vi "RT Main IMAQdx.vi"() -> ()   [LabVIEW 2017]
doc: "The myRIO Custom FPGA Project template acquires button data from the onboard button and displays the button value on a Boolean indicator. The SYS.RDY indicator shows the FPGA status."
uses:
  Controls/Image Size.ctl
  <vilib>/userdefined/High Color/IMAQdx.ctl
  <vilib>/FPGAPlugInAG/Dynamic/niLvFpga_Close_Dynamic.vi
  <vilib>/rvi/errors/niLvFpgaAdjustHostInterfaceError.vi
  <vilib>/Utility/error.llb/Error Cluster From Error Code.vi
  <vilib>/FPGAPlugInAG/Dynamic/niLvFpga_Run_Dynamic.vi
  <vilib>/myRIO/Common/Instrument Driver Framework/Utilities/vis/FPGA Ref Manager.vi
  <vilib>/myRIO/Common/Instrument Driver Framework/Utilities/vis/Ref Counter.vi
  <vilib>/rvi/interface/common/niFpgaCacheSessionInfoDynamic.vi
  <vilib>/rvi/interface/RandomDataEmulation/nirviRandomDataOpen.vi
  <vilib>/rvi/interface/nirviCloseFPGA/nirviCloseFPGA.xnode
  <vilib>/rvi/interface/nirviMethod/nirviMethod.xnode
  <vilib>/rvi/interface/nirviOpenFPGA/nirviOpenFPGA.xnode
  FPGA Main Image Processing.vi
  <vilib>/myRIO/Instrument Drivers/Utilities/Utilities.lvlib
  <vilib>/rvi/errors/niLvFpgaMergeErrorWithErrorCode.vi
  <vilib>/vision/NI_Vision_Development_Module.lvlib
  <vilib>/vision/driver/NI_Vision_Acquisition_Software.lvlib
  <vilib>/FPGAPlugInAG/Dynamic/niLvFpga_ReadFifo_Dynamic.vi
  <vilib>/FPGAPlugInAG/Dynamic/niLvFpga_WriteFifo_Dynamic.vi
  <vilib>/FPGAPlugInAG/Dynamic/niLvFpga_Reset_Dynamic.vi
  FPGA Bitfiles/SoCImageProcessi_FPGATarget_FPGAMainImagePro_62bwVpL48zU.lvbitx
  <vilib>/FPGAPlugInAG/myRIO-1900/niLvFpga_Open_myRIO-1900.vi
  <vilib>/rvi/interface/common/dynamic/niFpgaDynamicAddResources.vi
panel:
  out "Image Out":T1(plugin-control)
  out "Image In":T1(plugin-control)
  in  "Live":bool
  in  "Timeout":i32=2000
  out "FPS":dbl format="%#_3f"
  out "error out":errorcluster
  in  "Stop":bool
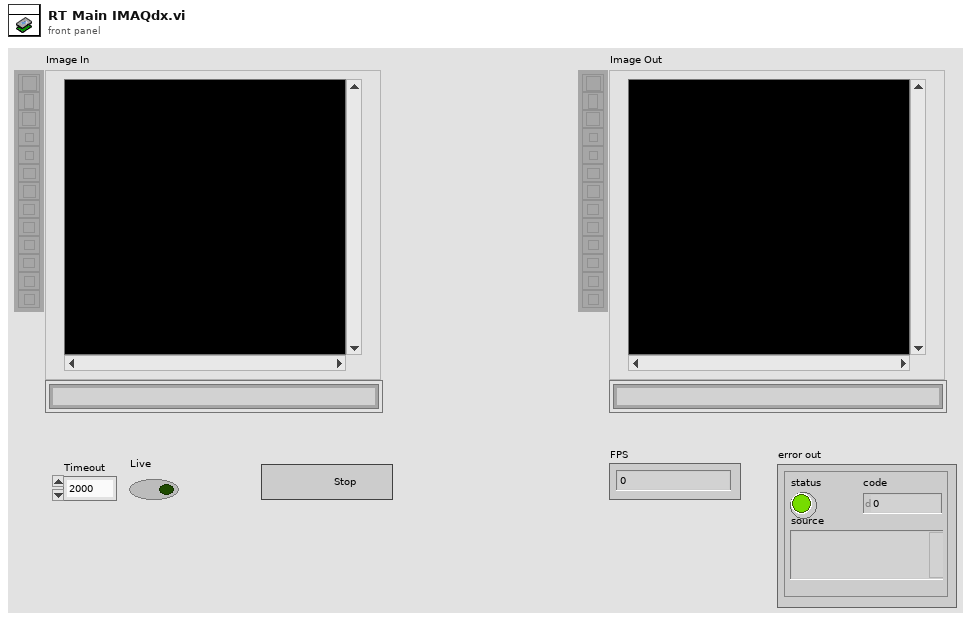
[diagram p1: front panel]
types:
  T1 = typedef "IMAQ Image.ctl" = refnum<image>
  T2 = typedef "Image Size.ctl" = cluster{"Rows (X)":u16, "Colums (Y)":u16}
  T3 = typedef "IMAQdx.ctl" = refnum<k21>
  T4 = typedef "Image Type" = u32
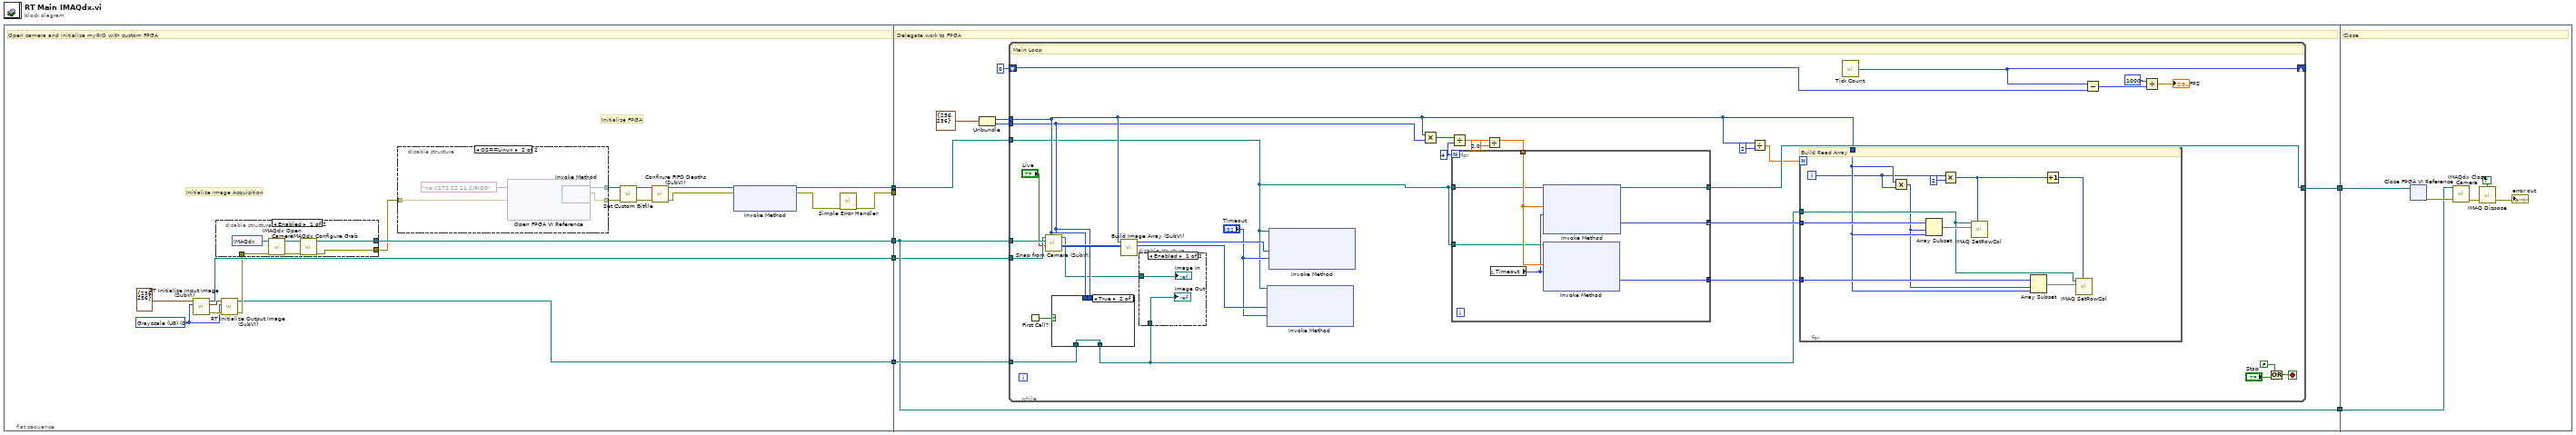
[diagram p0: block diagram]
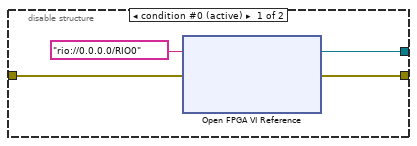
[diagram p3: hidden frame]
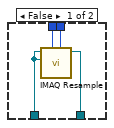
[diagram p5: hidden frame]
diagram:
  n1 = flat-sequence {
    tunnel: [w19] -> w7
    tunnel: [w24] -> w5
    tunnel: [w23] -> w4
    tunnel: [w9] -> w3
    tunnel: [w8] -> w1
    tunnel: w7 -> [w46]
    tunnel: [w50] -> w6
    tunnel: w5 -> [w44]
    tunnel: w4 -> [w43]
    tunnel: w3 -> [_]
    tunnel: [w44] -> w2
    tunnel: w1 -> [w45]
    tunnel: w6 -> [w114]
    tunnel: w2 -> [w109]
    frame #0 {
      w20 = T4 0 items=["Grayscale (U8)", "Grayscale (I16)", "Grayscale (SGL)", "Complex (CSG)", "RGB (U32)", "HSL (U32)", "RGB (U64)", "Grayscale (U16)"] ("Image Type")
      # "Initialize FPGA"
      # "Initialize Image Acquisition"
      # "Open camera and initialize myRIO with custom FPGA"
      n2 = call "RT Initialize Input Image (SubVI).vi"("Image Type"=w20, "Image Size In"=T2 {"Rows (X)"=256, "Colums (Y)"=256} ("Image Size")) -> ("error out"=w22:errorcluster, "Input Image Size Out"=w18:T2, "Input Image Out"=w23:T1)  [unwired: 7 in]
      n3 = call "RT Initialize Output Image (SubVI).vi"("error in (no error)"=w22, "Image Type"=w20, "Image Size In"=w18) -> ("error out"=w21:errorcluster, "Output Image Out"=w19:T1)  [unwired: 7 in]
      n4 = disable-structure shown="Enabled" {
        disable-tunnel: [w28 _] -> w24
        disable-tunnel: w21 -> [w27 w32]
        disable-tunnel: [w26 w32] -> w16
        frame Enabled {
          n5 = call <vilib>:"IMAQdx Open Camera.vi"("error in"=w27, "Session In"=T3 "cam0") -> ("error out"=w30:errorcluster, "Session Out"=w29:T3)  [unwired: 8 in]
          n6 = call <vilib>:"IMAQdx Configure Grab.vi"("error in"=w30, "Session In"=w29) -> ("error out"=w26:errorcluster, "Session Out"=w28:T3)  [unwired: 8 in]
        }
        frame Disabled {
        }
      }
      n7 = disable-structure shown="OS==Linux" {
        disable-tunnel: [w35 w39] -> w25
        disable-tunnel: [w34 w40] -> w17
        disable-tunnel: w16 -> [w33 w41]
        frame condition #0 (active) {
          n8 = xnode "Open FPGA VI Reference"("error in"=w33, "resource name"=tag "rio://0.0.0.0/RIO0") -> ("FPGA VI Reference Out"=w34:refnum<k20>, "error out"=w35:errorcluster)
        }
        frame condition #1 {
          n9 = xnode "Open FPGA VI Reference"("error in"=w41, "resource name"=tag "rio://172.22.11.2/RIO0") -> ("FPGA VI Reference Out"=w38:refnum<k20>, "error out"=w37:errorcluster)
          n10 = xnode "Invoke Method"("FPGA VI Reference In"=w38, "error in"=w37) -> ("FPGA VI Reference Out"=w40:refnum<k20>, "error out"=w39:errorcluster)
        }
      }
      n11 = call <vilib>:"Set Custom Bitfile.vi"("error in (no error)"=w25, "Custom FPGA Reference In"=w17) -> ("error out"=w13:errorcluster, "Custom FPGA Reference Out"=w10:refnum<k20>)  [unwired: 8 in]
      n12 = call "Confirure FIFO Depths (SubVI).vi"("error in (no error)"=w13, "Refnum in"=w10) -> ("error out"=w11:errorcluster, "Refnum out"=w12:refnum<k20>)  [unwired: 4 in, 4 out]
      n13 = xnode "Invoke Method"("FPGA VI Reference In"=w12, "error in"=w11) -> ("FPGA VI Reference Out"=w8:refnum<k20>, "error out"=w15:errorcluster)  [unwired: 1 in]
      n14 = call <vilib>:"Simple Error Handler.vi"("error in (no error)"=w15) -> ("error out"=w9:errorcluster)  [unwired: 4 in, 4 out]
    }
    frame #1 {
      # "Delegate work to FPGA"
      n15 = Unbundle(T2 {"Rows (X)"=256, "Colums (Y)"=256} ("Image Size")) -> ("Rows (X)"=w48:u16, "Colums (Y)"=w47:u16)
      n16 = while {
        shift-right: [w81] -> _
        shift-left: u32 0 ("Tick Count(mSec)") -> [w80]
        tunnel: [w76] -> w50
        tunnel: w48 -> [w59]
        tunnel: w47 -> [w58]
        tunnel: w45 -> [w52]
        tunnel: w44 -> [w66]
        tunnel: w46 -> [w57]
        tunnel: w43 -> [w65]
        stop <- w82 stop-if-true
        w72 = 4
        # "Main Loop"
        n17 = First Call?() -> (First Call?: T/F=w56:bool)
        n18 = call "Snap from Camera (SubVI).vi"("Colums (Y)"=w58, "Rows (X)"=w59, "Live"="Live", "Session In"=w66, "Image in"=w65) -> ("Image Pixels (U8)"=w64:u8[][], "Image out"=w55:T1)  [unwired: 3 in, 2 out]
        n19 = case shown="True" w56 {
          tunnel: w59 -> [w89 _]
          tunnel: w58 -> [w88 _]
          tunnel: w57 -> [w87 w90]
          tunnel: [w86 w90] -> w54
          frame False {
            n20 = call "IMAQ Resample"("X Resolution"=w88, "Y Resolution"=w89, "Image Dst"=w87, "Image Src"=w87) -> ("Image Dst Out"=w86:T1)  [unwired: 6 in, 1 out]
          }
          frame True {
          }
        }
        n21 = call "Build Image Array (SubVI).vi"("Image Pixels (U8) in"=w64, "Rows (X)"=w59) -> ("Image Pixels B (U8) 3"=w69:u8[], "Image Pixels A (U8) out"=w68:u8[])  [unwired: 8 in]
        n22 = disable-structure shown="Enabled" {
          disable-tunnel: w55 -> [w85 _]
          disable-tunnel: w54 -> [w84 _]
          frame Enabled {
            "Image In" <- w85
            "Image Out" <- w84
          }
          frame Disabled {
          }
        }
        n23 = xnode "Invoke Method"("FPGA VI Reference In"=w52, "Data"=w69, "Timeout (ms)"="Timeout") -> ()  [unwired: 1 in, 3 out]
        n24 = xnode "Invoke Method"("FPGA VI Reference In"=w52, "Data"=w68, "Timeout (ms)"="Timeout") -> ()  [unwired: 1 in, 3 out]
        n25 = Multiply(x=w59, y=w58) -> (x*y=w73:u32)
        n26 = Divide(x=w73, y=w72) -> (x/y=w74:dbl)
        n27 = Divide(x=w74, y=2.0) -> (x/y=w71:dbl)
        n28 = for {
          N: w72 -> [_]
          tunnel: w71 -> [w108]
          tunnel: [w107] -> w77 mode=concatenating
          tunnel: [w105] -> w75 mode=concatenating
          tunnel: w52 -> [w104]
          tunnel: [w106] -> w76
          tunnel: w52 -> [w102]
          n29 = local read "Timeout"() -> (w103:i32)
          n30 = xnode "Invoke Method"("FPGA VI Reference In"=w102, "Number of Elements"=w108, "Timeout (ms)"=w103) -> ("Data"=w107:u8[])  [unwired: 1 in, 3 out]
          n31 = xnode "Invoke Method"("FPGA VI Reference In"=w104, "Number of Elements"=w108, "Timeout (ms)"=w103) -> ("FPGA VI Reference Out"=w106:refnum<k20>, "Data"=w105:u8[])  [unwired: 1 in, 2 out]
        }
        n32 = Divide(x=w59, y=u16 2) -> (x/y=w60:dbl)
        n33 = for {
          N: w60 -> [_]
          tunnel: w77 -> [w101]
          tunnel: w75 -> [w100]
          tunnel: w54 -> [w96]
          tunnel: w59 -> [w97]
          i -> [w95]
          # "Build Read Array"
          n34 = Multiply(x=w97, y=w95) -> (x*y=w94:i32)
          n35 = Array Subset(array=w100, index=w94, length=w97) -> (w99:u8[])
          n36 = Multiply(x=w95, y=2) -> (x*y=w92:i32)
          n37 = call "IMAQ SetRowCol"("Number"=w92, "Pixels (U8)"=w99, "Image"=w96) -> ()  [unwired: 7 in, 2 out]
          n38 = Array Subset(array=w101, index=w94, length=w97) -> (w98:u8[])
          n39 = Increment(x=w92) -> (x+1=w91:i32)
          n40 = call "IMAQ SetRowCol"("Number"=w91, "Pixels (U8)"=w98, "Image"=w96) -> ()  [unwired: 7 in, 2 out]
        }
        n41 = call "Tick Count"() -> ("Tick Count(mSec)"=w81:u32)
        n42 = Subtract(x=w81, y=w80) -> (x-y=w79:u32)
        n43 = Divide(x=u32 1000, y=w79) -> (x/y=→"FPS":dbl)
        n44 = Or(x=FALSE, y="Stop") -> (x .or. y?=w82:bool)
      }
    }
    frame #2 {
      # "Close"
      n45 = xnode "Close FPGA VI Reference"("FPGA VI Reference In"=w114) -> ("error out"=w111:errorcluster)  [unwired: 1 in]
      n46 = call <vilib>:"IMAQdx Close Camera.vi"("error in"=w111, "Session In"=w109) -> ("error out"=w110:errorcluster)  [unwired: 9 in]
      n47 = call "IMAQ Dispose"("All Images? (No)"=TRUE, "error in (no error)"=w110) -> ("error out"=→"error out":errorcluster)  [unwired: 4 in]
    }
  }
